vi "GetIdInSN.vi"(11 "sn":string) -> (3 "id":string)   [LabVIEW 2012]
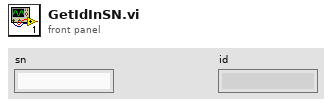
[diagram p1: front panel]
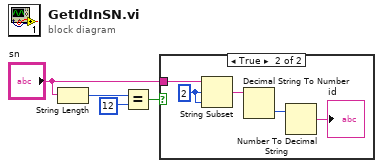
[diagram p0: block diagram]
diagram:
  n1 = String Length(string="sn") -> (length=w4:i32)
  n2 = Equal?(x=w4, y=12) -> (x = y?=w2:bool)
  n3 = case shown="True" w2 {
    tunnel: "sn" -> [_ w6]
    frame False {
    }
    frame True {
      w5 = 2
      n4 = String Subset(string=w6, offset (0)=w5, length (rest)=w5) -> (substring=w7:string)
      n5 = Decimal String To Number(string=w7) -> (number=w8:i32)  [unwired: 2 in, 1 out]
      n6 = Number To Decimal String(number=w8) -> (decimal integer string=→"id":string)  [unwired: 1 in]
    }
  }
